vi "01AMT800_GetNext.vi"(7 "Pattern":T1(array[ring]), 8 "error in (no error)":errorcluster, 10 "Value":i32, 11 "Enum":T2(ring)) -> (0 "error out":errorcluster, 3 "String":string)   [LabVIEW 2015]
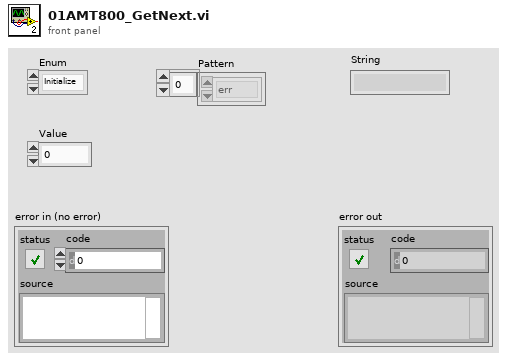
[diagram p1: front panel]
types:
  T1 = enum16{"err", "mph:", "inc:", "cnfg:", "loop:", "type", "ver", "part:", "led2:", "xmph", "led1", "ptmp", "mtmp", "vbus", "iamp", "vin", "amps", "RSET", "ramp:", "res:", "rng:", "rpm", "vbat", "lift"}[]
  T2 = enum16{"Initialize", "Next", "Send RSET", "Set MPH", "Set INC", "Part to 0", "Get MPH", "Set RES", "Set RAMP"}
  T3 = enum16{"err", "mph:", "inc:", "cnfg:", "loop:", "type", "ver", "part:", "led2:", "xmph", "led1", "ptmp", "mtmp", "vbus", "iamp", "vin", "amps", "RSET"}[]
  T4 = cluster{"Pattern":enum16{"err", "mph:", "inc:", "cnfg:", "loop:", "type", "ver", "part:", "led2:", "xmph", "led1", "ptmp", "mtmp", "vbus", "iamp", "vin", "amps", "RSET", "ramp:", "res:", "rng:", "rpm", "vbat", "lift"}[], "Index":i32, "mph":i32, "inc":i32, "part":i32, "ramp":i32, "res":i32}
  T5 = enum16{"err", "mph:", "inc:", "cnfg:", "loop:", "type", "ver", "part:", "led2:", "xmph", "led1", "ptmp", "mtmp", "vbus", "iamp", "vin", "amps", "RSET"}
  T6 = enum16{"err", "mph:", "inc:", "cnfg:", "loop:", "type", "ver", "part:", "led2:", "xmph", "led1", "ptmp", "mtmp", "vbus", "iamp", "vin", "amps", "RSET", "ramp:", "res:", "rng:", "rpm", "vbat", "lift"}
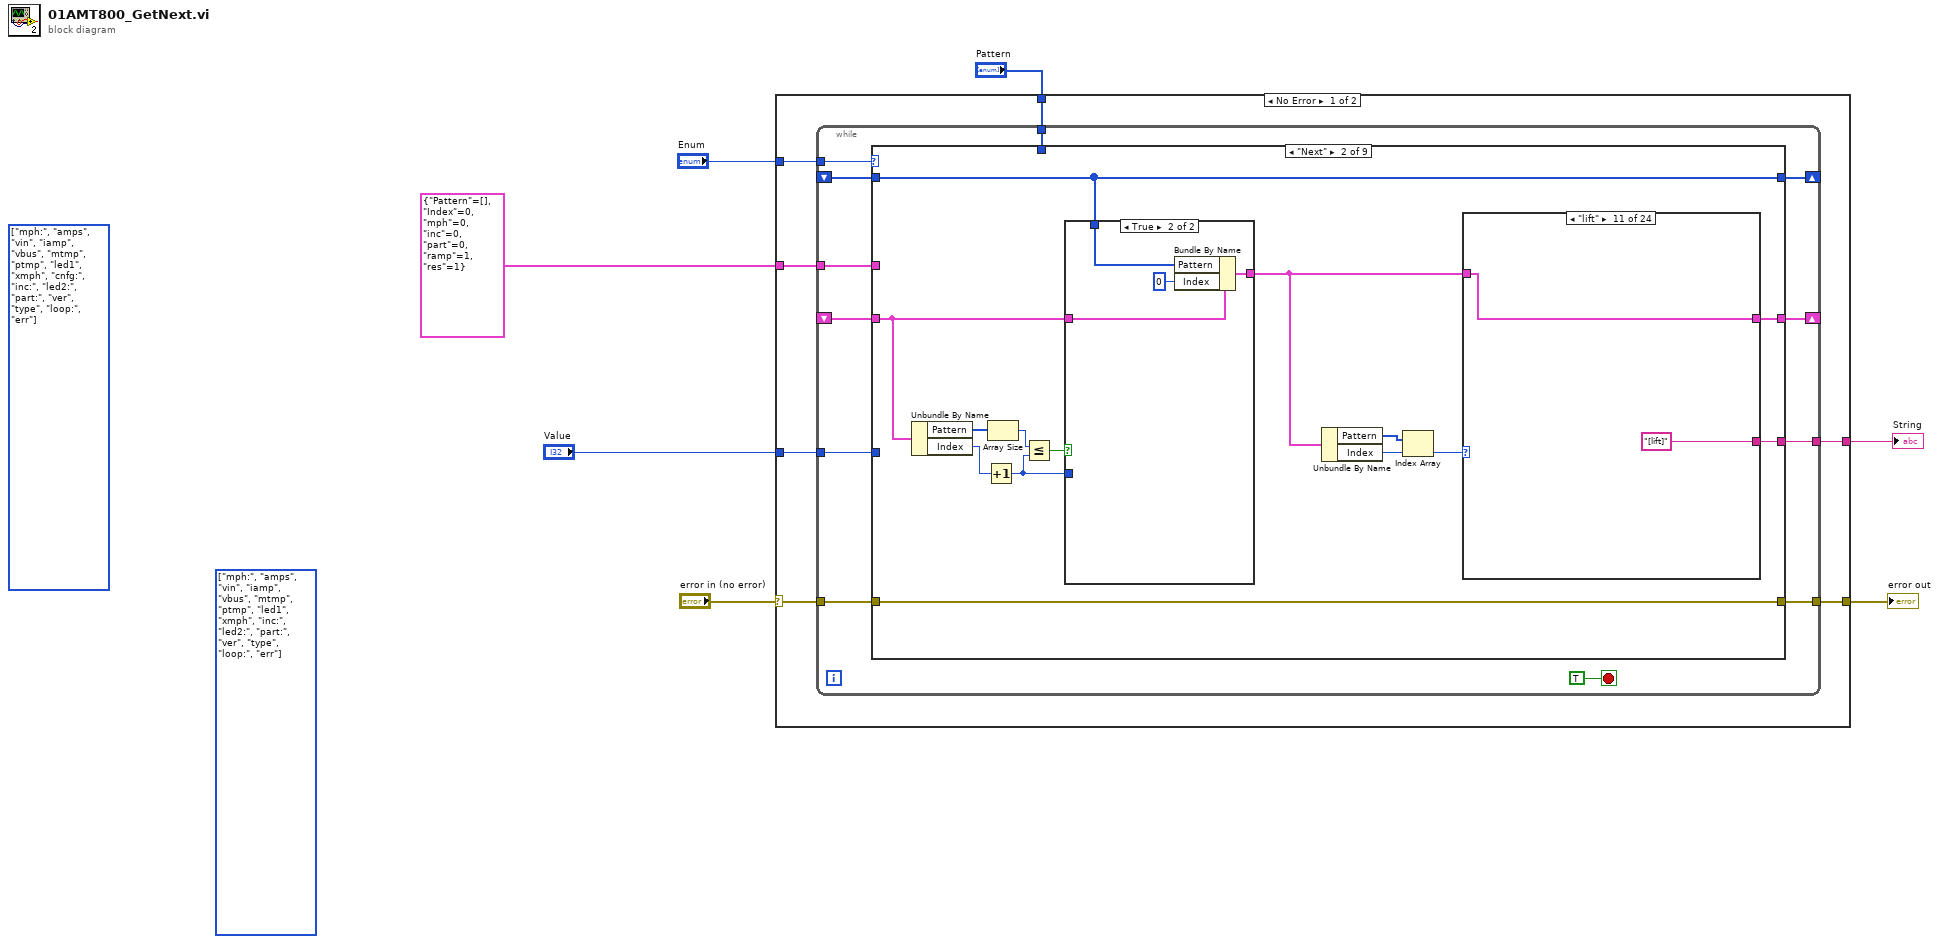
[diagram p0: block diagram]
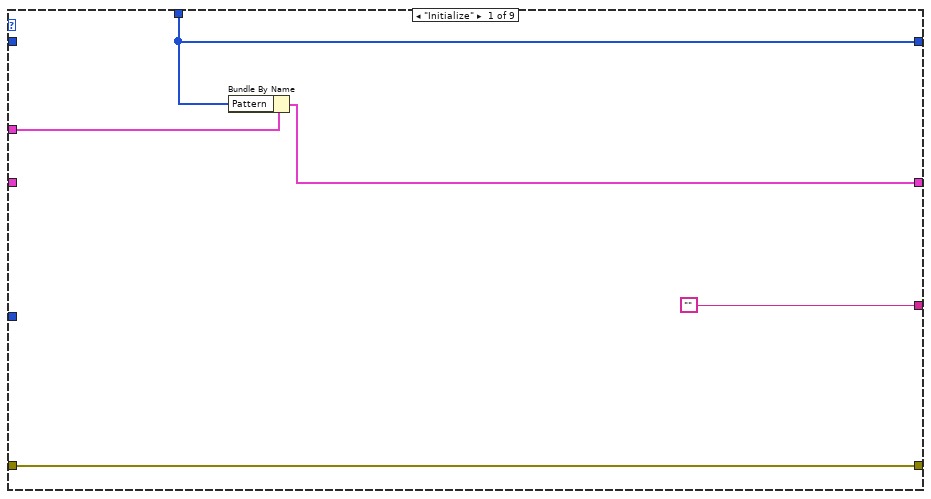
[diagram p2: hidden frame]
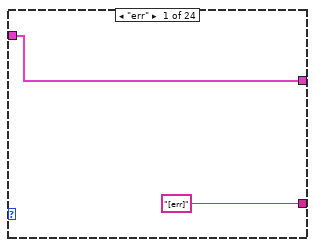
[diagram p3: hidden frame]
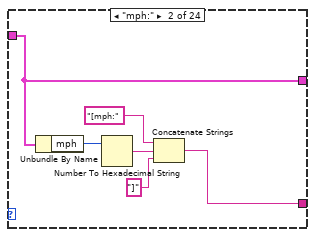
[diagram p4: hidden frame]
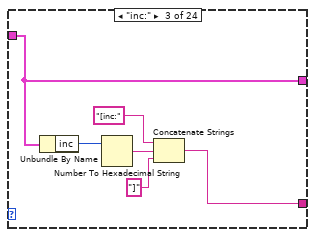
[diagram p5: hidden frame]
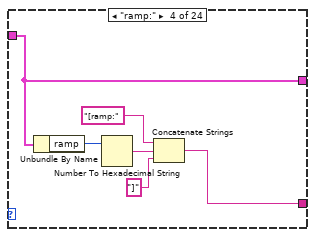
[diagram p6: hidden frame]
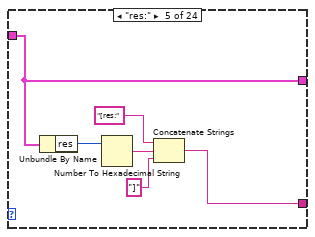
[diagram p7: hidden frame]
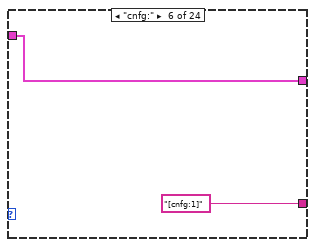
[diagram p8: hidden frame]
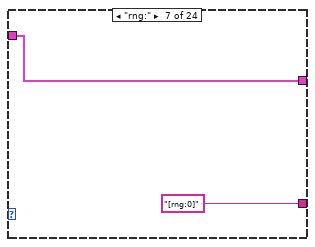
[diagram p9: hidden frame]
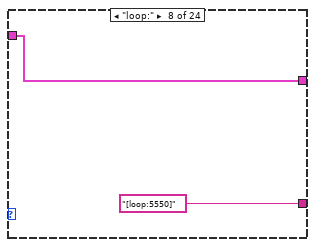
[diagram p10: hidden frame]
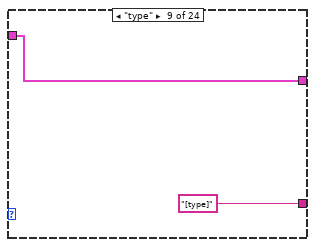
[diagram p11: hidden frame]
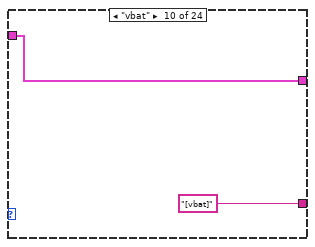
[diagram p12: hidden frame]
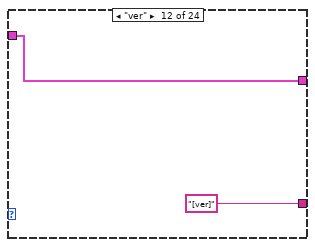
[diagram p13: hidden frame]
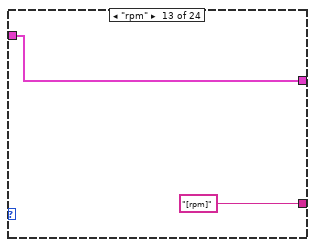
[diagram p14: hidden frame]
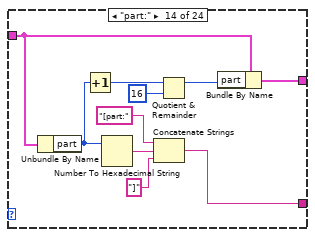
[diagram p15: hidden frame]
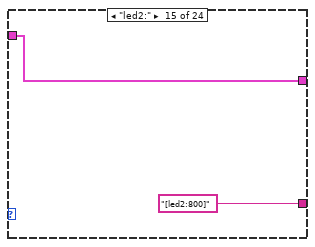
[diagram p16: hidden frame]
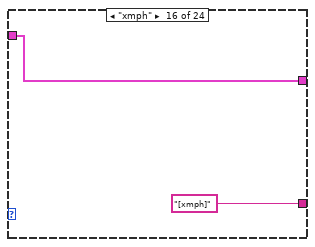
[diagram p17: hidden frame]
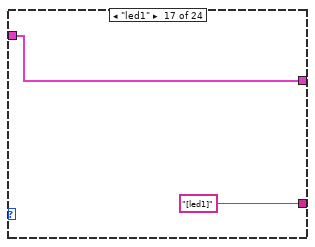
[diagram p18: hidden frame]
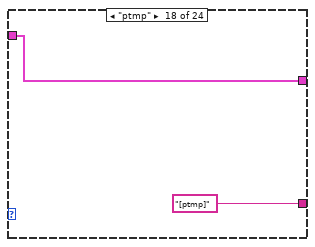
[diagram p19: hidden frame]
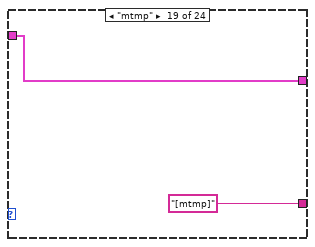
[diagram p20: hidden frame]
diagram:
  (unwired) T3 [enum."mph:", enum."amps", enum."vin", enum."iamp", enum."vbus", enum."mtmp", enum."ptmp", enum."led1", enum."xmph", enum."inc:", enum."led2:", enum."part:", enum."ver", enum."type", enum."loop:", enum."err"] items=["err", "mph:", "inc:", "cnfg:", "loop:", "type", "ver", "part:", "led2:", "xmph", "led1", "ptmp", "mtmp", "vbus", "iamp", "vin", "amps", "RSET"] ("Pattern")
  (unwired) T3 [enum."mph:", enum."amps", enum."vin", enum."iamp", enum."vbus", enum."mtmp", enum."ptmp", enum."led1", enum."xmph", enum."cnfg:", enum."inc:", enum."led2:", enum."part:", enum."ver", enum."type", enum."loop:", enum."err"] items=["err", "mph:", "inc:", "cnfg:", "loop:", "type", "ver", "part:", "led2:", "xmph", "led1", "ptmp", "mtmp", "vbus", "iamp", "vin", "amps", "RSET"] ("Pattern")
  n1 = case shown="No Error" "error in (no error)" {
    selector: "error in (no error)" -> [w14 w177]
    tunnel: [w11 w177] -> w6
    tunnel: [w13 ""] -> w5
    tunnel: "Enum" -> [w12 _]
    tunnel: T4 {"Pattern"=[], "Index"=0, "mph"=0, "inc"=0, "part"=0, "ramp"=1, "res"=1} -> [w10 _]
    tunnel: "Value" -> [w9 _]
    tunnel: "Pattern" -> [w8 _]
    frame No Error {
      n2 = while {
        tunnel: w14 -> [w23]
        tunnel: [w24] -> w13
        tunnel: w12 -> [w25]
        tunnel: [w22] -> w11
        tunnel: w10 -> [w21]
        shift-right: [w20] -> _
        shift-left: _ -> [w19]
        tunnel: w9 -> [w18]
        tunnel: w8 -> [w17]
        shift-right: [w16] -> _
        shift-left: _ -> [w15]
        stop <- TRUE stop-if-true
        n3 = case shown="\"Next\"" w25 {
          tunnel: ["" w35 "" "" "" "" w157 "" ""] -> w24
          tunnel: w23 -> [w30 w45 w132 w143 w149 w155 w163 w169 w175]
          tunnel: [w30 w45 w132 w143 w149 w155 w163 w169 w175] -> w22
          tunnel: w21 -> [w29 _ _ _ _ _ _ _ _]
          tunnel: [w28 w33 w133 w141 w147 w153 w158 w167 w173] -> w20
          tunnel: w19 -> [_ w39 w136 w142 w148 w154 w158 w168 w174]
          tunnel: w18 -> [_ _ _ w140 w146 _ _ w166 w172]
          tunnel: w17 -> [w27 _ _ _ _ _ _ _ _]
          tunnel: [w27 w32 w130 w138 w144 w150 w156 w164 w170] -> w16
          tunnel: w15 -> [_ w32 w130 w138 w144 w150 w156 w164 w170]
          frame "Initialize" {
            n4 = Bundle By Name(cluster=w29, "Pattern"=w27) -> (w28:T4)
          }
          frame "Next" {
            n5 = Unbundle By Name(w39) -> ("Pattern"=w44:T1, "Index"=w43:i32)
            n6 = Increment(x=w43) -> (x+1=w40:i32)
            n7 = Array Size(array=w44) -> (size(s)=w42:i32)
            n8 = Less Or Equal?(x=w42, y=w40) -> (x <= y?=w41:bool)
            n9 = case shown="True" w41 {
              tunnel: w40 -> [w124 _]
              tunnel: w39 -> [w125 w129]
              tunnel: [w123 w128] -> w34
              tunnel: w32 -> [_ w126]
              frame False {
                n10 = Bundle By Name(cluster=w125, "Index"=w124) -> (w123:T4)
              }
              frame True {
                n11 = Bundle By Name(cluster=w129, "Pattern"=w126, "Index"=0) -> (w128:T4)
              }
            }
            n12 = Unbundle By Name(w34) -> ("Pattern"=w37:T1, "Index"=w38:i32)
            n13 = Index Array(array=w37, index=w38) -> (element=w36:T6)
            n14 = case shown="\"lift\"" w36 {
              tunnel: ["[err]" w48 w54 w60 w66 "[cnfg:1]" "[rng:0]" "[loop:5550]" "[type]" "[vbat]" "[lift]" "[ver]" "[rpm]" w94 "[led2:800]" "[xmph]" "[led1]" "[ptmp]" "[mtmp]" "[vbus]" "[iamp]" "[vin]" "[amps]" "[RSET]"] -> w35
              tunnel: w34 -> [w46 w53 w59 w65 w71 w72 w74 w76 w79 w81 w83 w85 w87 w92 w99 w101 w103 w105 w107 w109 w111 w113 w115 w120]
              tunnel: [w46 w53 w59 w65 w71 w72 w74 w76 w79 w81 w83 w85 w87 w93 w99 w101 w103 w105 w107 w109 w111 w113 w115 w121] -> w33
              frame "err" {
              }
              frame "mph:" {
                n15 = Unbundle By Name(w53) -> ("mph"=w52:i32)
                n16 = Number To Hexadecimal String(2:w52) -> (0:w51:string)  [unwired: 1 in]
                n17 = Concatenate Strings("[mph:" ("string"), w51, "]" ("string")) -> (w48:string)
              }
              frame "inc:" {
                n18 = Unbundle By Name(w59) -> ("inc"=w58:i32)
                n19 = Number To Hexadecimal String(2:w58) -> (0:w57:string)  [unwired: 1 in]
                n20 = Concatenate Strings("[inc:" ("string"), w57, "]" ("string")) -> (w54:string)
              }
              frame "ramp:" {
                n21 = Unbundle By Name(w65) -> ("ramp"=w64:i32)
                n22 = Number To Hexadecimal String(2:w64) -> (0:w63:string)  [unwired: 1 in]
                n23 = Concatenate Strings("[ramp:" ("string"), w63, "]" ("string")) -> (w60:string)
              }
              frame "res:" {
                n24 = Unbundle By Name(w71) -> ("res"=w70:i32)
                n25 = Number To Hexadecimal String(2:w70) -> (0:w69:string)  [unwired: 1 in]
                n26 = Concatenate Strings("[res:" ("string"), w69, "]" ("string")) -> (w66:string)
              }
              frame "cnfg:" {
              }
              frame "rng:" {
              }
              frame "loop:" {
              }
              frame "type" {
              }
              frame "vbat" {
              }
              frame "lift" {
              }
              frame "ver" {
              }
              frame "rpm" {
              }
              frame "part:" {
                n27 = Unbundle By Name(w92) -> ("part"=w91:i32)
                n28 = Increment(x=w91) -> (x+1=w90:i32)
                n29 = Number To Hexadecimal String(2:w91) -> (0:w97:string)  [unwired: 1 in]
                n30 = Concatenate Strings("[part:" ("string"), w97, "]" ("string")) -> (w94:string)
                n31 = Quotient & Remainder(x=w90, y=16) -> (x-y*floor(x/y)=w89:i32)  [unwired: 1 out]
                n32 = Bundle By Name(cluster=w92, "part"=w89) -> (w93:T4)
              }
              frame "led2:" {
              }
              frame "xmph" {
              }
              frame "led1" {
              }
              frame "ptmp" {
              }
              frame "mtmp" {
              }
              frame "vbus" {
              }
              frame "iamp" {
              }
              frame "vin" {
              }
              frame "amps" {
              }
              frame "RSET" {
                n33 = Bundle By Name(cluster=w120, "mph"=0, "inc"=0, "ramp"=1, "res"=1) -> (w121:T4)
              }
            }
          }
          frame "Send RSET" {
            n34 = Unbundle By Name(w136) -> ("Pattern"=w135:T1)
            n35 = Build Array (concatenate)(w135, T5."RSET") -> (w134:T1)
            n36 = Bundle By Name(cluster=w136, "Pattern"=w134) -> (w133:T4)
          }
          frame "Set MPH" {
            n37 = Bundle By Name(cluster=w142, "mph"=w140) -> (w141:T4)
          }
          frame "Set INC" {
            n38 = Bundle By Name(cluster=w148, "inc"=w146) -> (w147:T4)
          }
          frame "Part to 0" {
            n39 = Bundle By Name(cluster=w154, "part"=0) -> (w153:T4)
          }
          frame "Get MPH" {
            n40 = Unbundle By Name(w158) -> ("mph"=w159:i32)
            n41 = Number To Hexadecimal String(2:w159) -> (0:w160:string)  [unwired: 1 in]
            n42 = Concatenate Strings("[mph:" ("string"), w160, "]" ("string")) -> (w157:string)
          }
          frame "Set RES" {
            n43 = Bundle By Name(cluster=w168, "res"=w166) -> (w167:T4)
          }
          frame "Set RAMP" {
            n44 = Bundle By Name(cluster=w174, "ramp"=w172) -> (w173:T4)
          }
        }
      }
    }
    frame Error {
    }
  }
  "error out" <- w6
  "String" <- w5
